vi "Conveyer Belt speed control.vi"(1 "Conveyer Belt Info":T1) -> (0 "Conveyer Belt Info out":T1)   [LabVIEW 2012]
uses:
  Conveyer Belt Global Data.vi
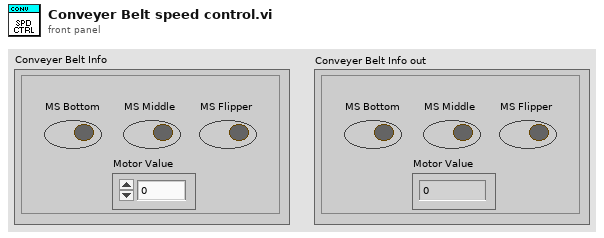
[diagram p1: front panel]
types:
  T1 = cluster{"MS Bottom":bool, "MS Middle":bool, "MS Flipper":bool, "Motor Value":dbl}
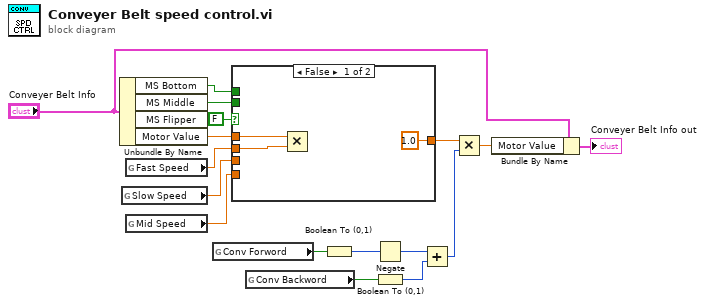
[diagram p0: block diagram]
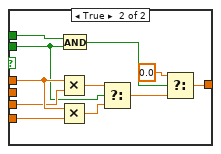
[diagram p2: hidden frame]
diagram:
  n1 = Unbundle By Name("Conveyer Belt Info") -> ("MS Bottom"=w10:bool, "MS Middle"=w12:bool, "Motor Value"=w15:dbl)  [unwired: 1 out]
  n2 = global read "Conveyer Belt Global Data.vi" "Slow Speed"() -> (w11:dbl)
  n3 = global read "Conveyer Belt Global Data.vi" "Fast Speed"() -> (w14:dbl)
  n4 = global read "Conveyer Belt Global Data.vi" "Mid Speed"() -> (w13:dbl)
  n5 = global read "Conveyer Belt Global Data.vi" "Conv Forword"() -> (w3:bool)
  n6 = case shown="False" FALSE {
    tunnel: w15 -> [w20 w29]
    tunnel: w14 -> [w19 _]
    tunnel: [1.0 ("t") w26] -> w5
    tunnel: w13 -> [_ w31]
    tunnel: w12 -> [_ w23]
    tunnel: w11 -> [_ w28]
    tunnel: w10 -> [_ w24]
    frame False {
      n7 = Multiply(x=w20, y=w19) -> ()  [unwired: 1 out]
    }
    frame True {
      n8 = Multiply(x=w29, y=w28) -> (x*y=w27:dbl)
      n9 = Multiply(x=w29, y=w31) -> (x*y=w30:dbl)
      n10 = And(x=w24, y=w23) -> (x .and. y?=w25:bool)
      n11 = Select(t=w27, s=w23, f=w30) -> (s? t:f=w21:dbl)
      n12 = Select(t=0.0, s=w25, f=w21) -> (s? t:f=w26:dbl)
    }
  }
  n13 = global read "Conveyer Belt Global Data.vi" "Conv Backword"() -> (w2:bool)
  n14 = Boolean To (0,1)(Boolean=w3) -> (0, 1=w8:i16)
  n15 = Negate(x=w8) -> (-x=w7:i16)
  n16 = Boolean To (0,1)(Boolean=w2) -> (0, 1=w9:i16)
  n17 = Add(x=w7, y=w9) -> (x+y=w4:i16)
  n18 = Multiply(x=w5, y=w4) -> (x*y=w6:dbl)
  n19 = Bundle By Name(cluster="Conveyer Belt Info", "Motor Value"=w6) -> (→"Conveyer Belt Info out":T1)
